vi "FindTopAndBottomEdges (SubVI).vi"(0 "Calibrated Image Array":T5[](array[typedef]), 1 "Fit Options":T10={"Number of Lines"=1, "Type"=enum."First Edge Rake", "Min. Score"=10.0, "Max. Score"=1000.0, "Orientation"=0.0, "Angle Range"=45.0, "Angle Tolerance"=1.0, "Step Size"=196, "Min. SNR (db)"=0.0, "Min. Points (%)"=25.0, "Hough Iterations"=5} {"Min. Points (%)" min=0.0 max=100.0; "Min. SNR (db)" min=0.0; "Max. Score" min=0.0 max=1024.0; "Min. Score" min=0.0 max=1024.0 step=1.0}, 5 "Options: Top Edge Search":T9={"Search Direction"=2, "Edge Options"={"Edge Polarity"=0, "Kernel Size"=5, "Width"=3, "Minimum Edge Strength"=16.0, "Interpolation Type"=enum."Bilinear Fixed", "Data Processing Method"=enum."Average"}, "Show Search Area"=TRUE, "Show Search Lines"=TRUE, "Show Edges Found"=TRUE, "Show Result"=TRUE, "Search Area Color"=65280, "Search Lines Color"=255, "Edge Locations Color"=16776960, "Result Color"=16711680, "Overlay Group Name"=""} {"Search Direction" items=["Left to Right", "Right to Left", "Top to Bottom", "Bottom to Top"]; "Edge Options"."Edge Polarity" items=["All Edges", "Rising Edges", "Falling Edges"]; "Edge Options"."Minimum Edge Strength" format="%.2f"; "Edge Options"."Width" step=2; "Edge Options"."Kernel Size" step=2}, 9 "Options: Bottom Edge Search":T9={"Search Direction"=3, "Edge Options"={"Edge Polarity"=2, "Kernel Size"=9, "Width"=3, "Minimum Edge Strength"=17.0, "Interpolation Type"=enum."Bilinear Fixed", "Data Processing Method"=enum."Average"}, "Show Search Area"=TRUE, "Show Search Lines"=TRUE, "Show Edges Found"=TRUE, "Show Result"=TRUE, "Search Area Color"=65280, "Search Lines Color"=255, "Edge Locations Color"=16776960, "Result Color"=16711680, "Overlay Group Name"=""} {"Search Direction" items=["Left to Right", "Right to Left", "Top to Bottom", "Bottom to Top"]; "Edge Options"."Edge Polarity" items=["All Edges", "Rising Edges", "Falling Edges"]; "Edge Options"."Minimum Edge Strength" format="%.2f"; "Edge Options"."Width" step=2; "Edge Options"."Kernel Size" step=2}, 11 "error in (no error)":errorcluster) -> (4 "Analyzed Image Array":T5[](array[typedef]), 6 "Top Edges":T6(array[cluster]), 8 "Bottom Edges":T6(array[cluster]), 10 "Array of Edge Endpoint Arrays":sgl[][][](array[numeric]), 15 "error out":errorcluster)   [LabVIEW 2016]
uses:
  <vilib>/vision/Measure.llb/Straight Edge Options.ctl
  <vilib>/vision/Measure.llb/Straight Edge Process.ctl
  <vilib>/vision/Measure.llb/Edge Options.ctl
  <vilib>/vision/Measure.llb/Edge Polarity.ctl
  <vilib>/vision/Image Controls.llb/IMAQ Image.ctl
  <vilib>/vision/NI_Vision_Development_Module.lvlib
  <resource>/objmgr/IMAQImage.rc
panel:
  in  "Search Rect 2":T1={"Left"=0, "Top"=0, "Right"=2147483647, "Bottom"=2147483647, "Rotation"=0.0} {"Rotation" format="%.2f"; "Left" scale=0.0..1024.0; "Right" scale=0.0..1024.0}
  out "searchrect":T2
  in  "Search Rect":T1={"Left"=0, "Top"=0, "Right"=2147483647, "Bottom"=2147483647, "Rotation"=0.0} {"Rotation" format="%.2f"; "Left" scale=0.0..1024.0; "Right" scale=0.0..1024.0}
  in  "ROI Descriptor before matches":T3={"Global Rectangle"=[675, 567, 1751, 1642], "Contours"=[{"ID"=enum."External", "Type"=7, "Coordinates"=[1212, 1104, 85, 537, 0, 0]}]} {"Contours"."Type" items=["No Selection", "Point", "Line", "Rectangle", "Oval", "Polygon", "Freehand Region", "Annulus", "Unused2", "Unused3", "Broken Line", "Freehand Line", "Rotated Rectangle"]}
  in  "Pattern Match Settings":T4={"Algorithm"=2, "Number of Matches Requested"=1, "Minimum Match Score"=800.0, "SubPixel Accuracy"=TRUE, "Rotation Angle Ranges"=[], "Show Search Area"=FALSE, "Show Result"=TRUE} {"Rotation Angle Ranges"."End" format="%.1f"; "Rotation Angle Ranges"."Start" format="%.1f"; "Minimum Match Score" min=0 max=1000 format="%.2f"; "Number of Matches Requested" min=1; "Algorithm" items=["All", "Low Discrepancy Sampling", "Grayscale Value Pyramid", "Gradients Pyramid"]}
  out "Template Image":T5
  in  "ROI Descriptor - BOTTOM":T3={"Global Rectangle"=[0, 898, 2592, 1846], "Contours"=[{"ID"=enum."External", "Type"=12, "Coordinates"=[2, 898, 2591, 1846, 0]}]} {"Contours"."Type" items=["No Selection", "Point", "Line", "Rectangle", "Oval", "Polygon", "Freehand Region", "Annulus", "Unused2", "Unused3", "Broken Line", "Freehand Line", "Rotated Rectangle"]}
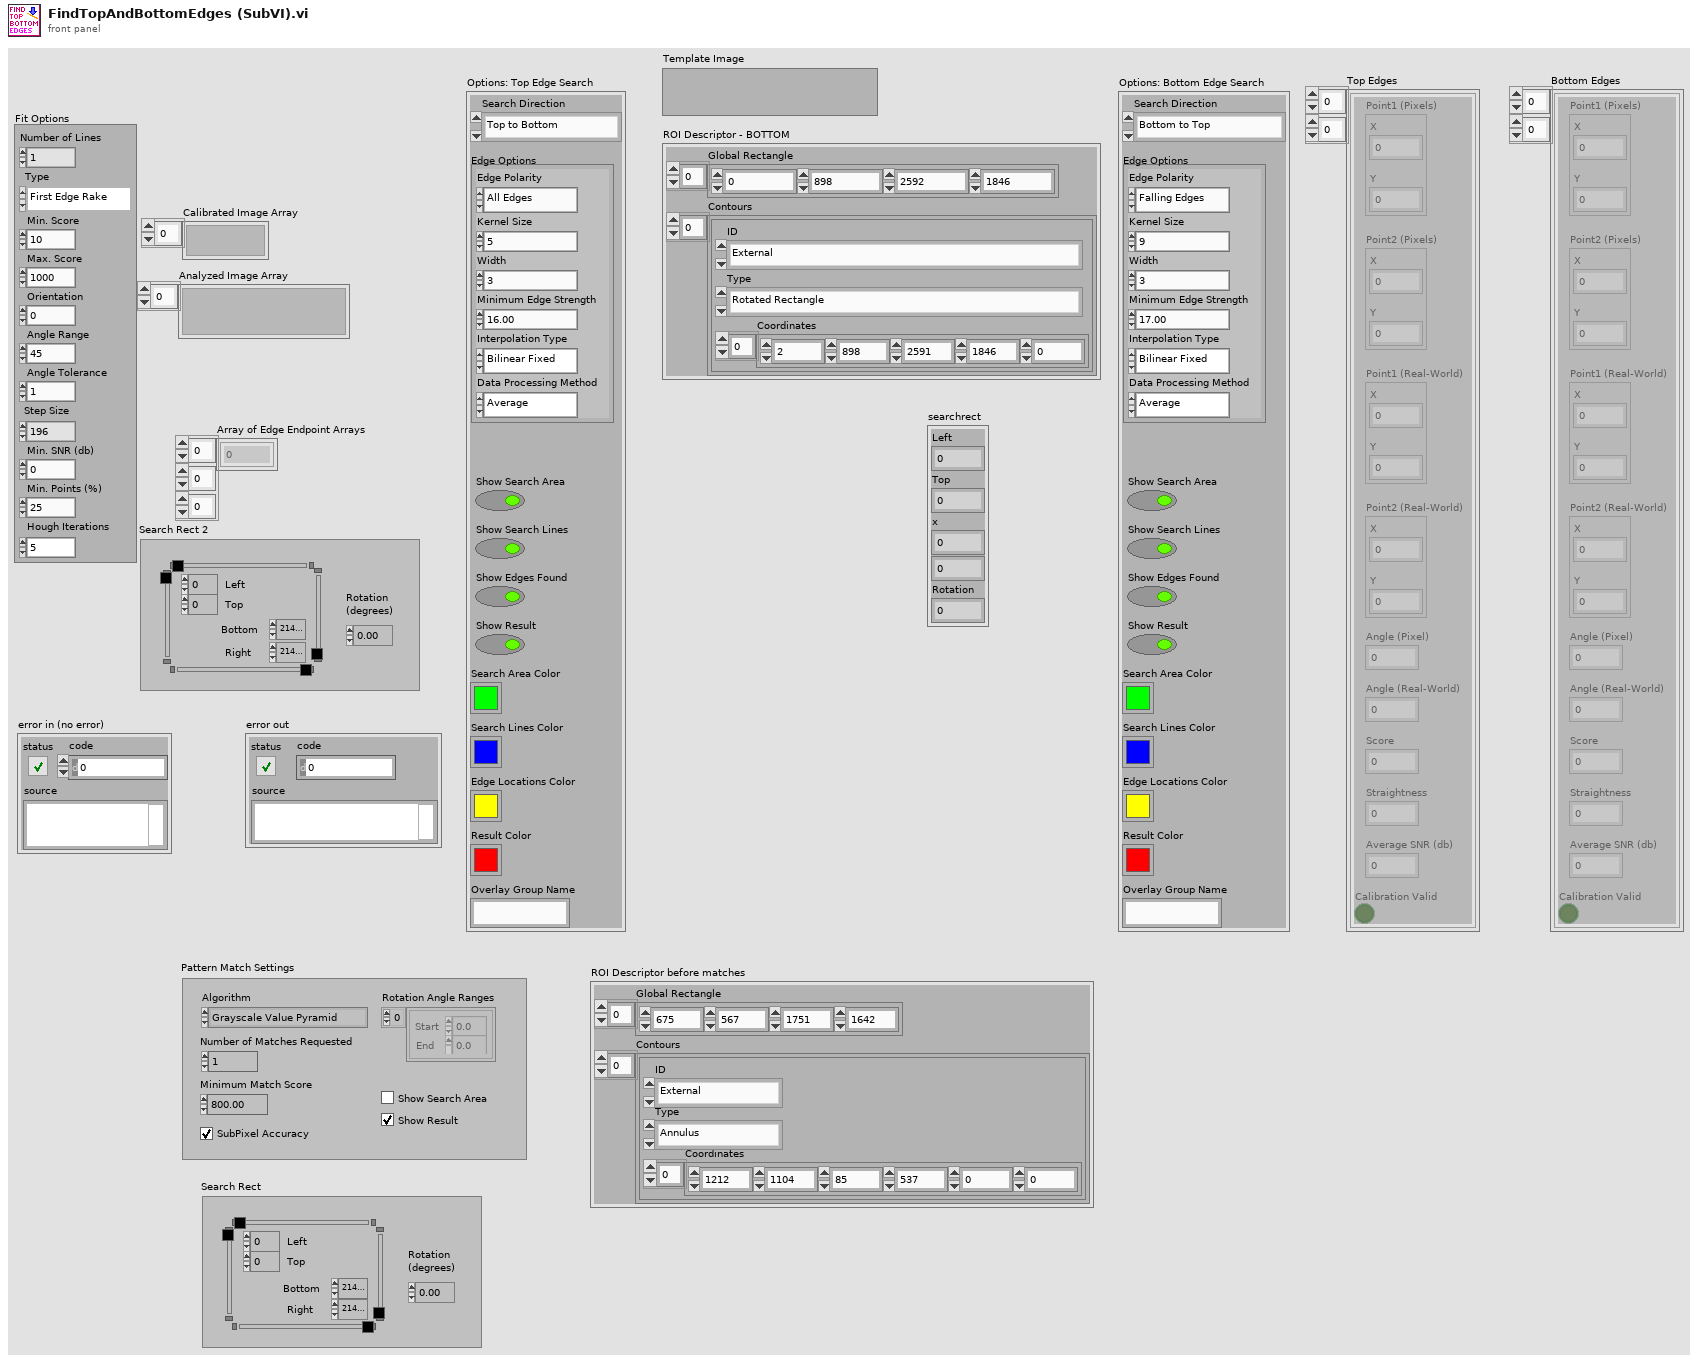
[diagram p1: front panel]
types:
  T1 = typedef "IMAQ Rectangle" = cluster{"Left":i32, "Top":i32, "Right":i32, "Bottom":i32, "Rotation":dbl}
  T2 = cluster{"Left":i32, "Top":i32, "x":i32, i32, "Rotation":dbl}
  T3 = cluster{"Global Rectangle":i32[], "Contours":cluster{"ID":enum32{"External", "Internal"}, "Type":u32, "Coordinates":i32[]}[]}
  T4 = cluster{"Algorithm":i32, "Number of Matches Requested":i32, "Minimum Match Score":sgl, "SubPixel Accuracy":bool, "Rotation Angle Ranges":cluster{"Start":sgl, "End":sgl}[], "Show Search Area":bool, "Show Result":bool}
  T5 = typedef "IMAQ Image.ctl" = refnum<image>
  T6 = cluster{"Point1 (Pixels)":cluster{"X":sgl, "Y":sgl}, "Point2 (Pixels)":cluster{"X":sgl, "Y":sgl}, "Point1 (Real-World)":cluster{"X":sgl, "Y":sgl}, "Point2 (Real-World)":cluster{"X":sgl, "Y":sgl}, "Angle (Pixel)":dbl, "Angle (Real-World)":dbl, "Score":dbl, "Straightness":dbl, "Average SNR (db)":dbl, "Calibration Valid":bool}[][]
  T7 = typedef "Edge Options.ctl" = cluster{"Edge Polarity":T8, "Kernel Size":u32, "Width":u32, "Minimum Edge Strength":sgl, "Interpolation Type":enum32{"Zero Order", "Bilinear", "Quadratic", "Cubic", "Bilinear Fixed"}, "Data Processing Method":enum32{"Average", "Median"}}
  T8 = typedef "Edge Polarity.ctl" = u32
  T9 = cluster{"Search Direction":u32, "Edge Options":T7, "Show Search Area":bool, "Show Search Lines":bool, "Show Edges Found":bool, "Show Result":bool, "Search Area Color":u32, "Search Lines Color":u32, "Edge Locations Color":u32, "Result Color":u32, "Overlay Group Name":string}
  T10 = typedef "Straight Edge Options.ctl" = cluster{"Number of Lines":i32, "Type":T11, "Min. Score":dbl, "Max. Score":dbl, "Orientation":dbl, "Angle Range":dbl, "Angle Tolerance":dbl, "Step Size":u32, "Min. SNR (db)":dbl, "Min. Points (%)":dbl, "Hough Iterations":i32}
  T11 = typedef "Straight Edge Process.ctl" = enum32{"First Edge Rake", "Best Edge Rake", "Hough Edge Rake", "First Edge Projection", "Best Edge Projection"}
  T12 = cluster{"Position":cluster{"x":sgl, "y":sgl}, "Angle":sgl, "Scale":sgl, "Score":sgl, "Bounding Box":cluster{"x":sgl, "y":sgl}[]}[]
  T13 = cluster{"Global Rectangle":i32[], cluster{"ID":enum32{"External", "Internal"}, "Type":u32, "Coordinates":i32[]}[]}
  T14 = cluster{"Point1 (Pixels)":cluster{"X":sgl, "Y":sgl}, "Point2 (Pixels)":cluster{"X":sgl, "Y":sgl}, "Point1 (Real-World)":cluster{"X":sgl, "Y":sgl}, "Point2 (Real-World)":cluster{"X":sgl, "Y":sgl}, "Angle (Pixel)":dbl, "Angle (Real-World)":dbl, "Score":dbl, "Straightness":dbl, "Average SNR (db)":dbl, "Calibration Valid":bool}[]
  T15 = cluster{"Point1 (Pixels)":cluster{"X":sgl, "Y":sgl}, "Point2 (Pixels)":cluster{"X":sgl, "Y":sgl}, "Point1 (Real-World)":cluster{"X":sgl, "Y":sgl}, "Point2 (Real-World)":cluster{"X":sgl, "Y":sgl}, "Angle (Pixel)":dbl, "Angle (Real-World)":dbl, "Score":dbl, "Straightness":dbl, "Average SNR (db)":dbl, "Calibration Valid":bool}
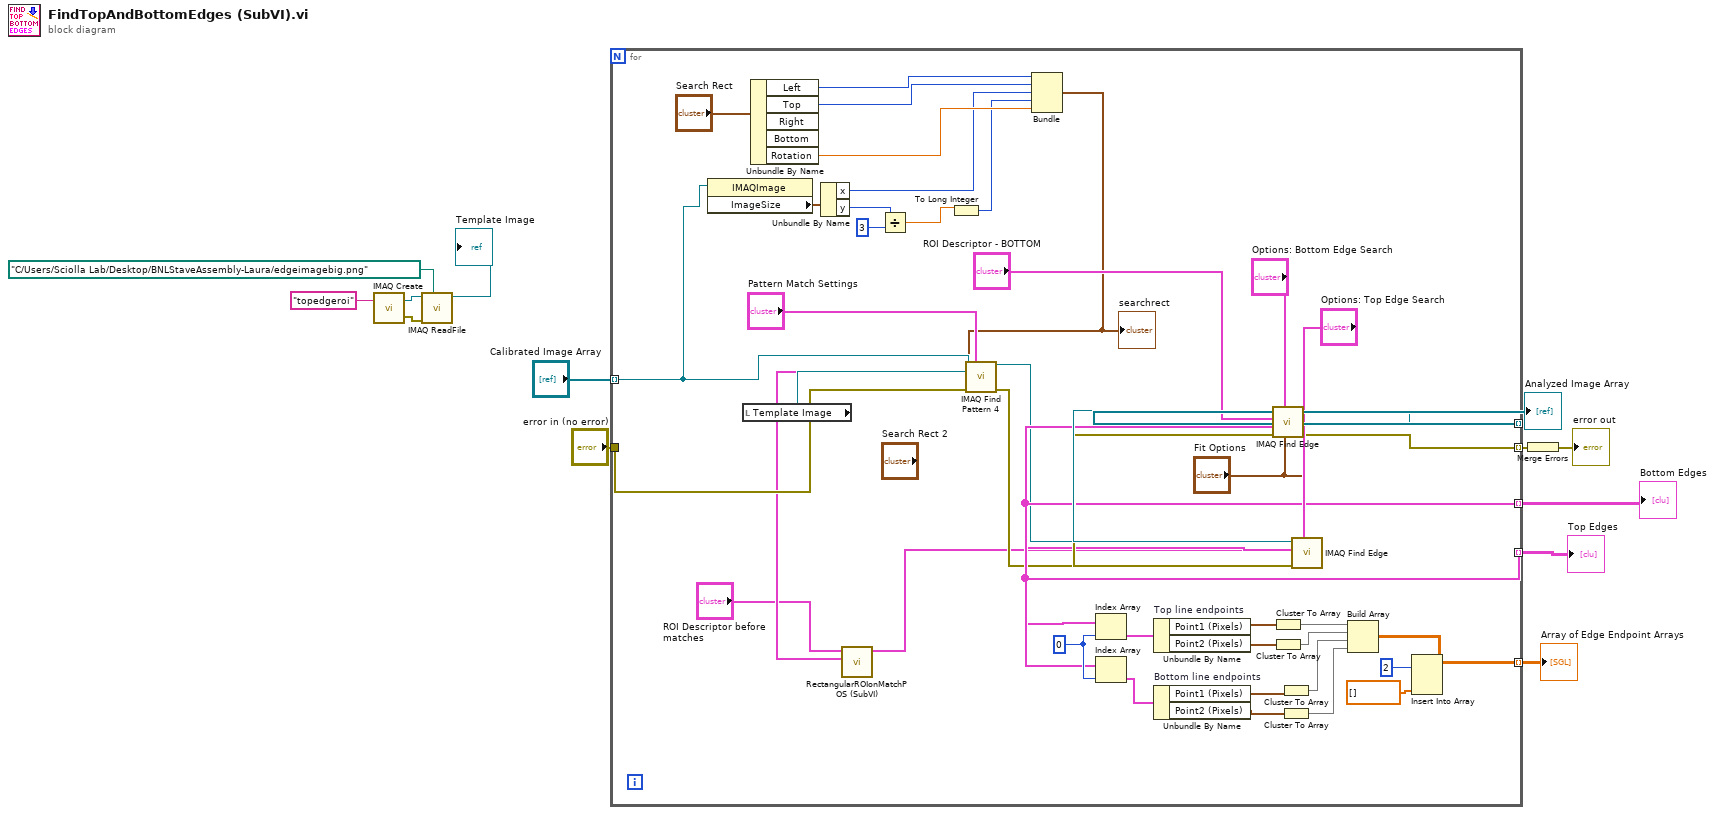
[diagram p0: block diagram]
diagram:
  n1 = call "IMAQ Create"("Image Name"="topedgeroi") -> ("New Image"=w3:T5, "error out"=w4:errorcluster)  [unwired: 4 in]
  n2 = call "IMAQ ReadFile"("File Path"=path "C:/Users/Sciolla Lab/Desktop/BNLStaveAssembly-Laura/edgeimagebig.png" ("Template File Path"), "error in (no error)"=w4, "Image"=w3) -> ("Image Out"=→"Template Image":T5)  [unwired: 4 in, 4 out]
  n3 = for {
    tunnel: "Calibrated Image Array" -> [w19] mode=indexing
    tunnel: "error in (no error)" -> [w33]
    tunnel: [w55] -> w10 mode=indexing
    tunnel: [w53] -> w13 mode=indexing
    tunnel: [w28] -> w8 mode=indexing
    tunnel: [w36] -> w7 mode=indexing
    tunnel: [w35] -> w6 mode=indexing
    w50 = 0 ("index")
    n4 = property class="IMAQImage"(reference=w19) -> ("ImageSize"=w21:cluster{"x":i32, "y":i32})  [unwired: 1 in, 2 out]
    n5 = local read "Template Image"() -> (w34:T5)
    n6 = Unbundle By Name("Search Rect") -> ("Left"=w24:i32, "Top"=w23:i32, "Rotation"=w22:dbl)  [unwired: 2 out]
    n7 = Unbundle By Name(w21) -> ("x"=w18:i32, "y"=w20:i32)
    n8 = Divide(x=w20, y=3) -> (x/y=w16:dbl)
    n9 = To Long Integer(number=w16) -> (32bit integer=w15:i32)
    n10 = Bundle("Left"=w24, "Top"=w23, "x"=w18, w15, "Rotation"=w22) -> (w14:T2)  [unwired: 1 in]
    "searchrect" <- w14
    n11 = call "IMAQ Find Pattern 4"("Image"=w19, "Template"=w34, "Search Rect"=w14, "error in"=w33, "Settings"="Pattern Match Settings") -> ("Image Out"=w31:T5, "Matches (pixel)"=w29:T12, "error out"=w32:errorcluster)  [unwired: 4 in, 4 out]
    n12 = call "RectangularROIonMatchPOS (SubVI).vi"("Matches (pixel)"=w29, "ROI Descriptor before matches"="ROI Descriptor before matches") -> ("ROI Descriptor after matches"=w26:T13)  [unwired: 9 in]
    n13 = call "IMAQ Find Edge"("Line Fit Options"="Fit Options", "Options"="Options: Top Edge Search", "error in (no error)"=w32, "ROI Descriptor"=w26, "Image"=w31) -> ("error out"=w51:errorcluster, "Straight Edges"=w28:T14, "Image Out"=w52:T5)  [unwired: 3 in, 1 out]
    n14 = Index Array(array=w28, index=w50) -> (element=w49:T15)
    n15 = Unbundle By Name "Top line endpoints"(w49) -> ("Point1 (Pixels)"=w47:cluster{"X":sgl, "Y":sgl}, "Point2 (Pixels)"=w46:cluster{"X":sgl, "Y":sgl})
    n16 = call "IMAQ Find Edge"("Line Fit Options"="Fit Options", "Options"="Options: Bottom Edge Search", "error in (no error)"=w51, "ROI Descriptor"="ROI Descriptor - BOTTOM", "Image"=w52) -> ("error out"=w55:errorcluster, "Straight Edges"=w36:T14, "Image Out"=w53:T5)  [unwired: 3 in, 1 out]
    n17 = Index Array(array=w36, index=w50) -> (element=w48:T15)
    n18 = Unbundle By Name "Bottom line endpoints"(w48) -> ("Point1 (Pixels)"=w39:cluster{"X":sgl, "Y":sgl}, "Point2 (Pixels)"=w40:cluster{"X":sgl, "Y":sgl})
    n19 = Cluster To Array(cluster=w47) -> (array=w45:sgl[])
    n20 = Cluster To Array(cluster=w46) -> (array=w44:sgl[])
    n21 = Cluster To Array(cluster=w39) -> (array=w38:sgl[])
    n22 = Cluster To Array(cluster=w40) -> (array=w37:sgl[])
    n23 = Build Array(w45, w44, w38, w37) -> (w43:sgl[][])
    n24 = Insert Into Array(array=w43, index (col)=2 ("disabled index (col)"), new element=sgl[] [] ("new element/subarray")) -> (w35:sgl[][])  [unwired: 1 in]
  }
  "Analyzed Image Array" <- w13
  "Top Edges" <- w8
  "Bottom Edges" <- w7
  "Array of Edge Endpoint Arrays" <- w6
  n25 = Merge Errors(w10) -> (→"error out":errorcluster)
